vi "Config Aout Limit.vi"(0 "VISA resource name":refnum<visa-resource-name>, 1 "Upper Capacitance (10.5 V)":dbl=10.5 min=-10.5 max=10.5 format="%#_6f", 2 "Lower Capacitance (-10.5 V)":dbl=-10.5 min=-10.5 max=10.5 format="%#_6f", 3 "Upper Loss (10.5 V)":dbl=10.5 min=-10.5 max=10.5 format="%#_6f", 4 "Lower Loss (-10.5 V)":dbl=-10.5 min=-10.5 max=10.5 format="%#_6f", 5 "error in":errorcluster) -> (14 "VISA resource name out":refnum<visa-resource-name>, 19 "error out":errorcluster)   [LabVIEW 2019, in "Andeen-Hagerling 2700(400 firmware).lvlib"]
doc: "Sets the upper and lower protection limits, respectively, of the capacitance and loss channel output voltages."
uses:
  Andeen-Hagerling 2700(400 firmware).lvlib
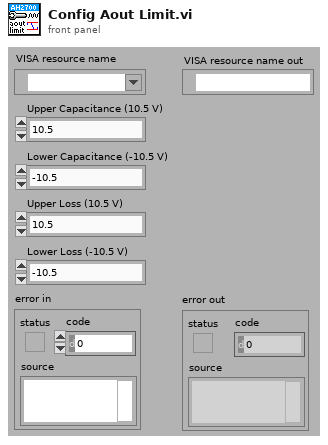
[diagram p1: front panel]
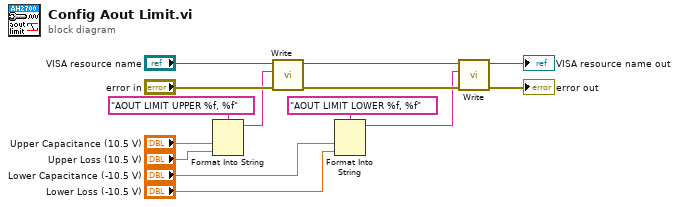
[diagram p0: block diagram]
diagram:
  n1 = Format Into String(format string="AOUT LIMIT UPPER %f, %f", "Upper Capacitance (10.5 V)", "Upper Loss (10.5 V)") -> (resulting string=w9:string)  [unwired: 2 in, 1 out]
  n2 = call "Write.vi"("error in"="error in", "command"=w9, "VISA resource name"="VISA resource name") -> ("error out"=w6:errorcluster, "VISA resource name out"=w8:refnum<visa-resource-name>)  [unwired: 7 in]
  n3 = Format Into String(format string="AOUT LIMIT LOWER %f, %f", "Lower Capacitance (-10.5 V)", "Lower Loss (-10.5 V)") -> (resulting string=w2:string)  [unwired: 2 in, 1 out]
  n4 = call "Write.vi"("error in"=w6, "command"=w2, "VISA resource name"=w8) -> ("error out"=→"error out":errorcluster, "VISA resource name out"=→"VISA resource name out":refnum<visa-resource-name>)  [unwired: 7 in]
